vi "rx_pduExtract.vi"(5 "output bit stream":i8[](array[numeric])) -> (0 "found?":bool, 1 "packet len":u32, 2 "ppdu":i8[](array[numeric]))   [LabVIEW 2014]
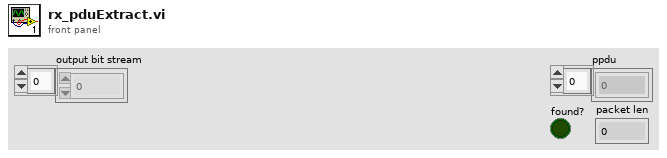
[diagram p1: front panel]
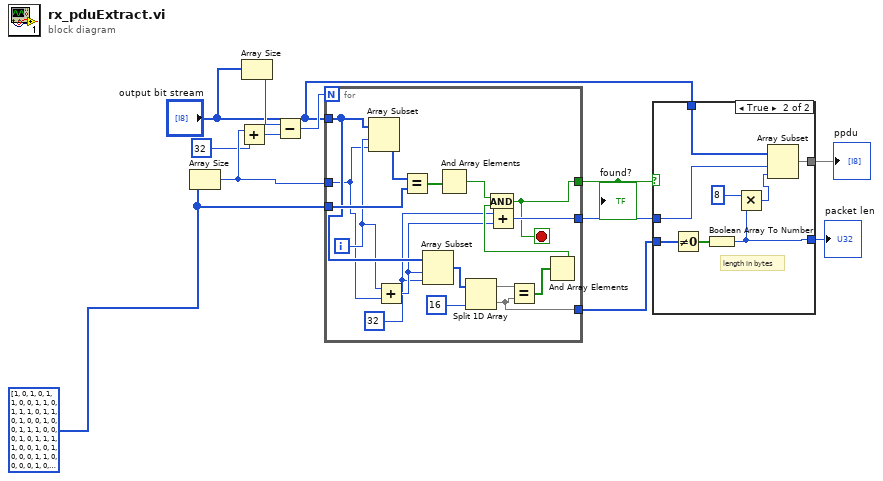
[diagram p0: block diagram]
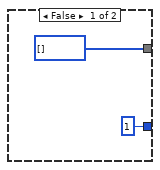
[diagram p2: hidden frame]
diagram:
  w1 = i16[] [1, 0, 1, 0, 1, 1, 0, 0, 1, 1, 0, 1, 1, 1, 0, 1, 1, 0, 1, 0, 0, 1, 0, 0, 1, 1, 1, 0, 0, 0, 1, 0, 1, 1, 1, 1, 0, 0, 1, 0, 1, 0, 0, 0, 1, 1, 0, 0, 0, 0, 1, 0, 0, 0, 0, 0, 1, 1, 1, 1, 1, 1, 0, 0] ("preamble(64) 2")
  n1 = Array Size(array=w1) -> (size(s)=w4:i32)
  n2 = Add(x=w4, y=32) -> (x+y=w5:i32)
  n3 = Array Size(array="output bit stream") -> (size(s)=w12:i32)
  n4 = Subtract(x=w12, y=w5) -> (x-y=w11:i32)
  n5 = for {
    N: w11 -> [_]
    tunnel: "output bit stream" -> [w25]
    tunnel: w4 -> [w23]
    tunnel: w1 -> [w28]
    tunnel: [w16] -> w10
    tunnel: [w26] -> w9
    tunnel: [w14] -> w6
    i -> [w24]
    stop <- w16 stop-if-true
    w13 = 32 ("length")
    n6 = Array Subset(array=w25, index=w24, length=w23) -> (w29:i8[])
    n7 = Add(x=w24, y=w23) -> (x+y=w15:i32)
    n8 = Equal?(x=w29, y=w28) -> (x = y?=w27:bool[])
    n9 = Array Subset(array=w25, index=w15, length=w13) -> (w22:i8[])
    n10 = And Array Elements(Boolean array=w27) -> (logical AND=w18:bool)
    n11 = Split 1D Array(array=w22, index=16) -> (first subarray=w20:i8[], second subarray=w14:i8[])
    n12 = Add(x=w13, y=w15) -> (x+y=w26:i32)
    n13 = Equal?(x=w20, y=w14) -> (x = y?=w19:bool[])
    n14 = And Array Elements(Boolean array=w19) -> (logical AND=w17:bool)
    n15 = And(x=w18, y=w17) -> (x .and. y?=w16:bool)
  }
  "found?" <- w10
  n16 = case shown="True" w10 {
    tunnel: w9 -> [_ w38]
    tunnel: "output bit stream" -> [_ w39]
    tunnel: [i8[] [] w37] -> w7
    tunnel: w6 -> [_ w36]
    tunnel: [u32 1 w32] -> w2
    frame False {
    }
    frame True {
      # "length in bytes"
      n17 = Not Equal To 0?(x=w36) -> (x != 0?=w35:bool[])
      n18 = Boolean Array To Number(Boolean array=w35) -> (number=w32:u32)
      n19 = Multiply(x=u32 8, y=w32) -> (x*y=w33:u32)
      n20 = Array Subset(array=w39, index=w38, length=w33) -> (w37:i8[])
    }
  }
  "ppdu" <- w7
  "packet len" <- w2
